vi "Chart Demo.vi"() -> ()   [LabVIEW 2021]
uses:
  Chart Actor Messages/Add Waveform to Chart Msg/Add Waveform to Chart Msg.lvclass/Add Waveform to Chart Msg.ctl
  <vilib>/ActorFramework/Message Enqueuer/Message Enqueuer.lvclass/Message Enqueuer.ctl
  <vilib>/ActorFramework/Message Enqueuer/Enqueue.vi
  Chart Actor/Chart Actor.lvclass
  C:/Program Files (x86)/National Instruments/LabVIEW 2021/vi.lib/ActorFramework/Actor/Actor.lvclass
  Chart Actor Messages/Add Waveform to Chart Msg/Add Waveform to Chart Msg.lvclass
  C:/Program Files (x86)/National Instruments/LabVIEW 2021/vi.lib/ActorFramework/Message/Message.lvclass
  <vilib>/ActorFramework/Stop Msg/Stop Msg.lvclass
  <vilib>/ActorFramework/Message Priority Queue/Priority Enqueue.vi
  <vilib>/measure/NI_MABase.lvlib
  <vilib>/ActorFramework/Actor/Actor.lvclass
panel:
  in  "amplitude":dbl=1.0 format="%0.2p"
  in  "stop":bool
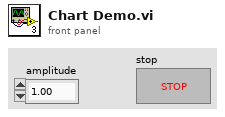
[diagram p1: front panel]
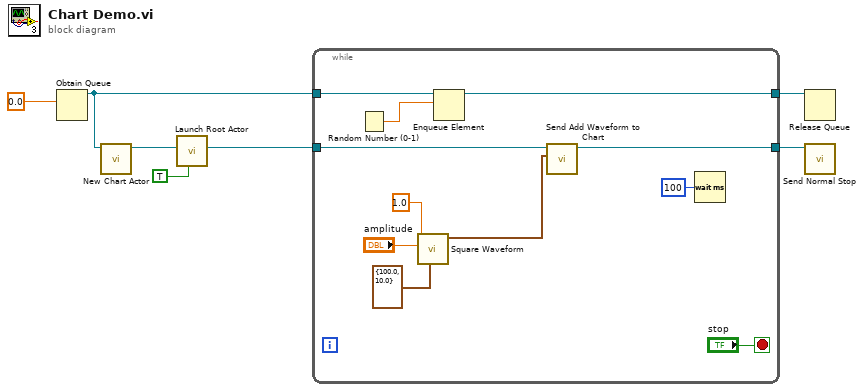
[diagram p0: block diagram]
diagram:
  n1 = Obtain Queue(element data type=0.0) -> (queue out=w2:refnum<queue>)  [unwired: 4 in, 2 out]
  n2 = call "New Chart Actor.vi"("Random Data Queue"=w2) -> ("Chart Actor out"=w3:refnum<class "Chart Actor.lvclass">)  [unwired: 9 in, 1 out]
  n3 = call <vilib>:"Launch Root Actor.vi"("Open Actor Core front panel? (F)"=TRUE, "Actor"=w3) -> ("Actor's Enqueuer"=w5:refnum<class "Message Enqueuer.lvclass">)  [unwired: 8 in, 1 out]
  n4 = while {
    tunnel: [w12] -> w6
    tunnel: w5 -> [w11]
    tunnel: w2 -> [w10]
    tunnel: [w8] -> w1
    stop <- "stop" stop-if-true
    n5 = Random Number (0-1)() -> (number: 0 to 1=w9:dbl)
    n6 = call <vilib>:"Square Waveform.vi"("sampling info"=cluster{"Fs":dbl, "#s":dbl} {"Fs"=100.0, "#s"=10.0}, "amplitude"="amplitude", "frequency"=1.0) -> ("signal out"=w13:waveform(dbl))  [unwired: 7 in, 1 out]
    n7 = Enqueue Element(queue=w10, element=w9) -> (queue out=w8:refnum<queue>)  [unwired: 2 in, 2 out]
    n8 = call "Send Add Waveform to Chart.vi"("Waveform In"=w13, "Message Enqueuer"=w11) -> ("Message Enqueuer out"=w12:refnum<class "Message Enqueuer.lvclass">)  [unwired: 8 in, 1 out]
    n9 = Wait (ms)(milliseconds to wait=u32 100) -> ()  [unwired: 1 out]
  }
  n10 = Release Queue(queue=w1) -> ()  [unwired: 2 in, 3 out]
  n11 = call <vilib>:"Send Normal Stop.vi"("Message Enqueuer"=w6) -> ()  [unwired: 10 in, 1 out]
